vi "set_config_cluster.vi"(8 "error in (no error)":errorcluster, 10 "config cluster variant":variant, 11 "ExperimentControllerDL090430DAQmxTriggered in":refnum<class "ExperimentControllerDL090430DAQmxTriggered.lvclass">) -> (0 "error out":errorcluster, 3 "ExperimentControllerDL090430DAQmxTriggered out":refnum<class "ExperimentControllerDL090430DAQmxTriggered.lvclass">)   [LabVIEW 2010, in "ExperimentControllerDL090430DAQmxTriggered.lvclass"]
uses:
  ExperimentControllerDL090430DAQmxTriggered.lvclass
  ExperimentControllerDL090430DAQmxTriggered.lvclass/ExperimentControllerDL090430DAQmxTriggered.ctl
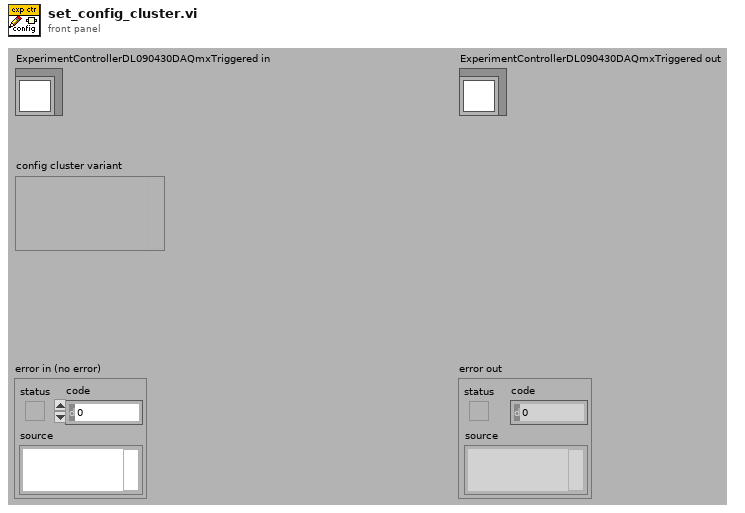
[diagram p1: front panel]
types:
  T1 = typedef "ExperimentControllerDL090430DAQmxTriggered.lvclass/config_data_cluster.ctl" = cluster{"trigger terminal":string, "trigger input line":string, "edge":i32, "mode":T2}
  T2 = typedef "ExperimentControllerDL090430DAQmxTriggered.lvclass/mode_enum.ctl" = enum16{"trigger", "gate"}
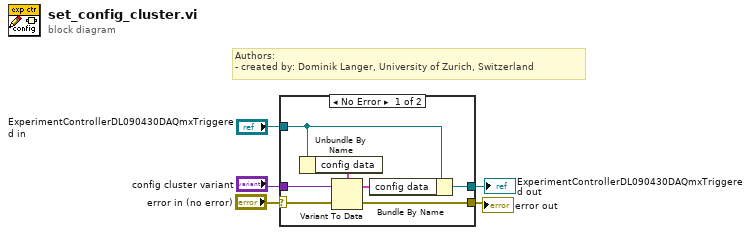
[diagram p0: block diagram]
diagram:
  # "Authors: \n- created by: Dominik Langer, University of Zurich, Switzerland"
  n1 = case shown="No Error" "error in (no error)" {
    selector: "error in (no error)" -> [w10 w13]
    tunnel: "ExperimentControllerDL090430DAQmxTriggered in" -> [w8 w14]
    tunnel: [w7 w13] -> w1
    tunnel: [w6 w14] -> w2
    tunnel: "config cluster variant" -> [w9 _]
    frame No Error {
      n2 = Unbundle By Name(w8) -> ("config data"=w12:T1)
      n3 = Variant To Data(error in=w10, Variant=w9, type=w12) -> (error out=w7:errorcluster, data=w11:T1)
      n4 = Bundle By Name(cluster=w8, "config data"=w11) -> (w6:refnum<class "ExperimentControllerDL090430DAQmxTriggered.lvclass">)
    }
    frame Error {
    }
  }
  "error out" <- w1
  "ExperimentControllerDL090430DAQmxTriggered out" <- w2
